vi "editgraficadora.vi"() -> ()   [LabVIEW 2020]
panel:
  out "Numeric":dbl
  in  "stop":bool
  out "Alarma":bool
  out "Waveform Chart":dynamicdata(graph)
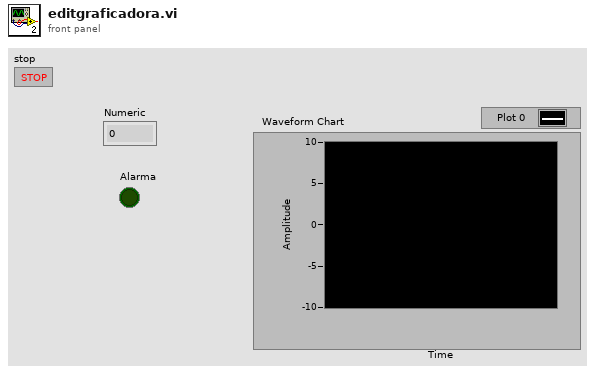
[diagram p1: front panel]
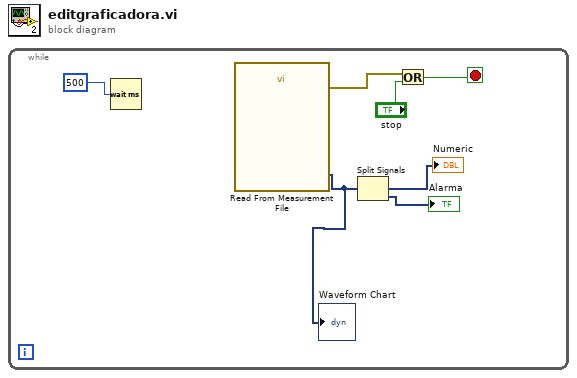
[diagram p0: block diagram]
diagram:
  n1 = while {
    stop <- w4 stop-if-true
    n2 = Wait (ms)(milliseconds to wait=500) -> ()  [unwired: 1 out]
    n3 = call "Read From Measurement File"() -> ("error out"=w5:errorcluster, "Signals"=w1:dynamicdata)  [unwired: 6 in, 4 out]
    "Waveform Chart" <- w1
    n4 = Split Signals(w1) -> (→"Numeric":dynamicdata, →"Alarma":dynamicdata)  [unwired: 3 in, 1 out]
    n5 = Or(x=w5, y="stop") -> (x .or. y?=w4:bool)
  }
